vi "Measurement B.vi"(0 "Inputs":T2, 7 "First name":string, 9 "Last name":string) -> (4 "Result":dbl, 8 "Name":T1, 10 "Full name":string)   [LabVIEW 2021]
uses:
  controls/Measurement Inputs.ctl
  Reusables/controls/Username.ctl
  controls/Offset value.ctl
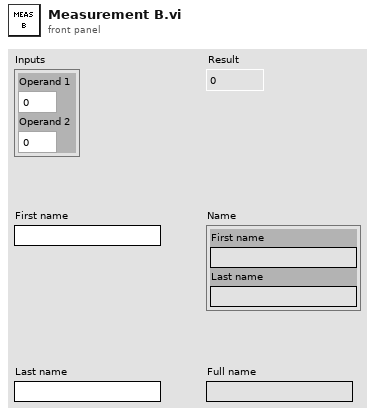
[diagram p1: front panel]
types:
  T1 = typedef "Username.ctl" = cluster{"First name":string, "Last name":string}
  T2 = typedef "Measurement Inputs.ctl" = cluster{"Operand 1":dbl, "Operand 2":dbl}
  T3 = typedef "Offset value.ctl" = cluster{"offset":dbl}
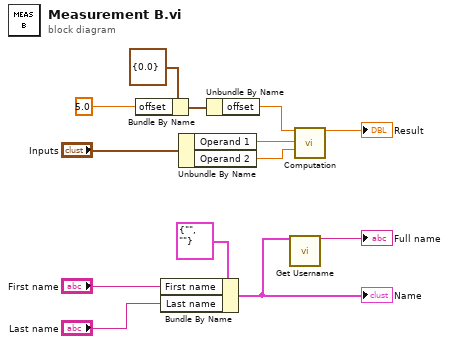
[diagram p0: block diagram]
diagram:
  n1 = Bundle By Name(cluster=T3 {"offset"=0.0}, "offset"=5.0) -> (w6:T3)
  n2 = Bundle By Name(cluster=T1 {"First name"="", "Last name"=""} ("Name"), "First name"="First name", "Last name"="Last name") -> (w2:T1)
  "Name" <- w2
  n3 = Unbundle By Name("Inputs") -> ("Operand 1"=w12:dbl, "Operand 2"=w11:dbl)
  n4 = Unbundle By Name(w6) -> ("offset"=w10:dbl)
  n5 = call "Get Username.vi"("Name"=w2) -> ("Full name"=→"Full name":string)  [unwired: 14 in]
  n6 = call "Computation.vi"("offset"=w10, "Operand 1"=w12, "Operand 2"=w11) -> ("Result"=→"Result":dbl)  [unwired: 12 in]
